vi "Measurement Termination In Progress.vi"() -> (3 "VI Path":path=path "C:/Users/ies-pg-8881/Documents/srd-adg-rf/src/fpt/Alpha_Demo/FPT Shared VIs/Termination In Progress.vi")   [LabVIEW 2023]
panel:
  out "Message 2":string="The measurement is being aborted. DO NOT start another measurement until this prompt is dismissed.\n\n"
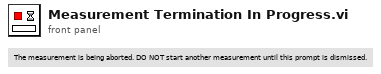
[diagram p1: front panel]
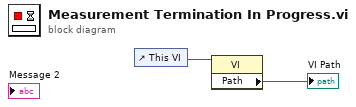
[diagram p0: block diagram]
diagram:
  n1 = control-ref of="This VI"() -> (w2:refnum<vi>)
  n2 = property class="VI"(reference=w2) -> ("Path"=→"VI Path":path)  [unwired: 1 in, 2 out]
